vi "CreateProtectedEvents.vi"(8 "error in (no error)":errorcluster, 11 "SMO":refnum<class "SMO.lvclass">) -> (0 "error out":errorcluster, 3 "SMO out":refnum<class "SMO.lvclass">)   [LabVIEW 2021, in "smo.lvlib" / "SMO.lvclass"]
uses:
  SMO.lvclass
  Typedefs/StopProcessEventData--Cluster.ctl
  Typedefs/AbortProcessEventData--Cluster.ctl
  Typedefs/SMO Dependency Event--Cluster.ctl
  Typedefs/SMO Dependency Event--Enum.ctl
  SMO.lvclass/SMO.ctl
panel:
  # "For instructions on how to use the JKI State Machine Objects, examples and video tutorials, visit:\nhttp://jki.net/state-machine-objects/\n\nJKI State Machine Objects™\nhttp://jki.net/state-machine-objects/\nCopyright (C) 2005-2015, JKI <info@jki.net>\nALL RIGHTS RESERVED"
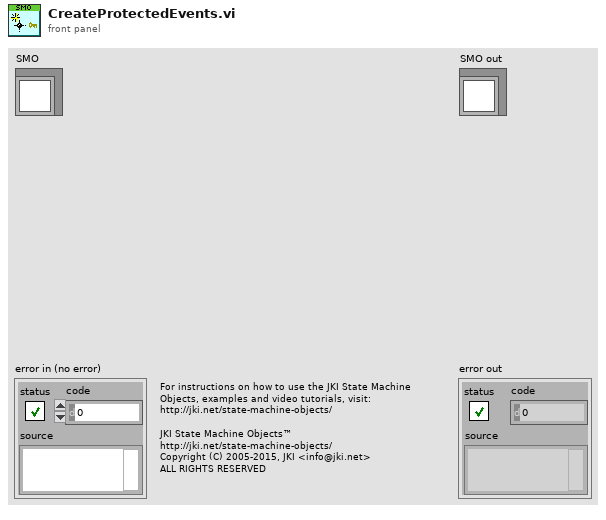
[diagram p1: front panel]
types:
  T1 = typedef "smo.lvlib/SMO.lvclass/SMO Dependency Event--Cluster.ctl" = cluster{"Name":string, "GUID":string, "Event":T2}
  T2 = typedef "smo.lvlib/SMO.lvclass/SMO Dependency Event--Enum.ctl" = enum16{"Added", "Removed", "Started", "Stopped"}
  T3 = typedef "smo.lvlib/SMO.lvclass/AbortProcessEventData--Cluster.ctl" = cluster{"Time Stamp":timestamp}
  T4 = typedef "smo.lvlib/SMO.lvclass/StopProcessEventData--Cluster.ctl" = cluster{"Time Stamp":timestamp}
  T5 = cluster{"Stop Processes":refnum<user-event>, "Abort Processes":refnum<user-event>, "Config Changed":refnum<user-event>, "Dependency Event":refnum<user-event>}
  T6 = typedef "smo.lvlib/SMO.lvclass/PrivateData--Ref.ctl" = refnum<data-value>
  T7 = typedef "smo.lvlib/SMO.lvclass/PrivateData--Cluster.ctl" = cluster{"Parent Call":T8, "Registered Processes":T9[], "Sync Notifier":refnum<notifier>, "Process Error Notifier":refnum<notifier>, "Protected Events":T10, "Public Events":T11, "SMO State":T12, "[Attributes]":variant, "Launcher Close":refnum<notifier>, "Caller Watchdog":refnum<queue>, "Accessibility":T13, "NbStaticDependencies":u32}
  T8 = typedef "smo.lvlib/SMO.lvclass/Parent Call--Enum.ctl" = enum16{"Allows parent to run", "Does not request parent to run"}
  T9 = typedef "smo.lvlib/SMO.lvclass/RegisteredProcessData--Cluster.ctl" = cluster{"Name":string, "Static VI Ref":refnum<vi>, "Running":bool, "NotifierRef":u32}
  T10 = typedef "smo.lvlib/SMO.lvclass/Protected Events.ctl" = cluster{"StopProcesses":refnum<user-event>, "AbortProcesses":refnum<user-event>, "Config Changed":refnum<user-event>, "Dependency":refnum<user-event>}
  T11 = typedef "smo.lvlib/SMO.lvclass/Public Events.ctl" = cluster{"Error":refnum<user-event>, "State":refnum<user-event>, "Reserve State":refnum<user-event>}
  T12 = typedef "smo.lvlib/SMO.lvclass/SMOState --Enum.ctl" = enum16{"unknown", "Created", "Started", "Stopped"}
  T13 = typedef "smo.lvlib/SMO.lvclass/Accessibility--Cluster.ctl" = cluster{"Lock Key":string, "Reserve State":T14}
  T14 = typedef "smo.lvlib/SMO.lvclass/Reserve State--Enum.ctl" = enum16{"Unreserved", "Reserved", "Self-locked"}
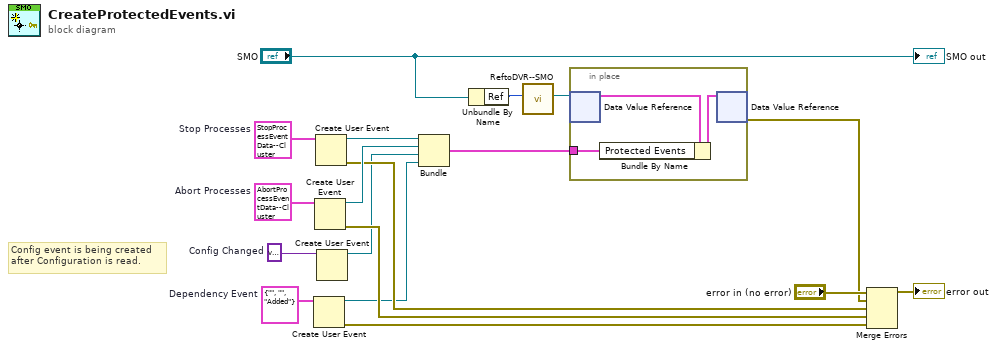
[diagram p0: block diagram]
diagram:
  w5 = variant  # Config Changed
  w8 = T1 {"Name"="", "GUID"="", "Event"=enum."Added"}  # Dependency Event
  w14 = T3 {"Time Stamp"=timestamp(0 s since 1904-01-01)}  # Abort Processes
  w15 = T4 {"Time Stamp"=timestamp(0 s since 1904-01-01)}  # Stop Processes
  # "Config event is being created\nafter Configuration is read."
  n1 = Create User Event(user event datatype=w8) -> (user event=w7:refnum<user-event>, error out=w6:errorcluster)  [unwired: 1 in]
  n2 = Create User Event(user event datatype=w14) -> (user event=w12:refnum<user-event>, error out=w9:errorcluster)  [unwired: 1 in]
  n3 = Create User Event(user event datatype=w15) -> (user event=w13:refnum<user-event>, error out=w10:errorcluster)  [unwired: 1 in]
  n4 = Create User Event(user event datatype=w5) -> (user event=w4:refnum<user-event>)  [unwired: 1 in, 1 out]
  n5 = Bundle("Stop Processes"=w13, "Abort Processes"=w12, "Config Changed"=w4, "Dependency Event"=w7) -> (w16:T5)  [unwired: 1 in]
  n6 = Unbundle By Name("SMO") -> ("Ref"=w3:u32)
  n7 = call "ReftoDVR--SMO.vi"("Ref"=w3) -> ("Ref"=w2:T6)  [unwired: 10 in]
  n8 = in-place {
    in-place-border: w16 -> [w19]
    n9 = in-place-dvr #1(w2) -> (w21:T7)  [unwired: 1 out]
    n10 = Bundle By Name(cluster=w21, "Protected Events"=w19) -> (w20:T7)
    n11 = in-place-dvr #1(w20) -> (w11:errorcluster)  [unwired: 1 out]
  }
  n12 = Merge Errors("error in (no error)", w11, w10, w9, w6) -> (→"error out":errorcluster)
  "SMO out" <- "SMO"
